vi "Reporte.vi"(10 "End Time":timestamp, 11 "Start Time":timestamp) -> ()   [LabVIEW 2020, in "UI.lvlib"]
uses:
  UI.lvlib
  Contabilidad/Contabilidad.lvlib
panel:
  out "Result Set":string[][](table) caption="Table Servicios"
  out "Tabla Servicios":string[](array[string])
  out "Ganacia Total":dbl
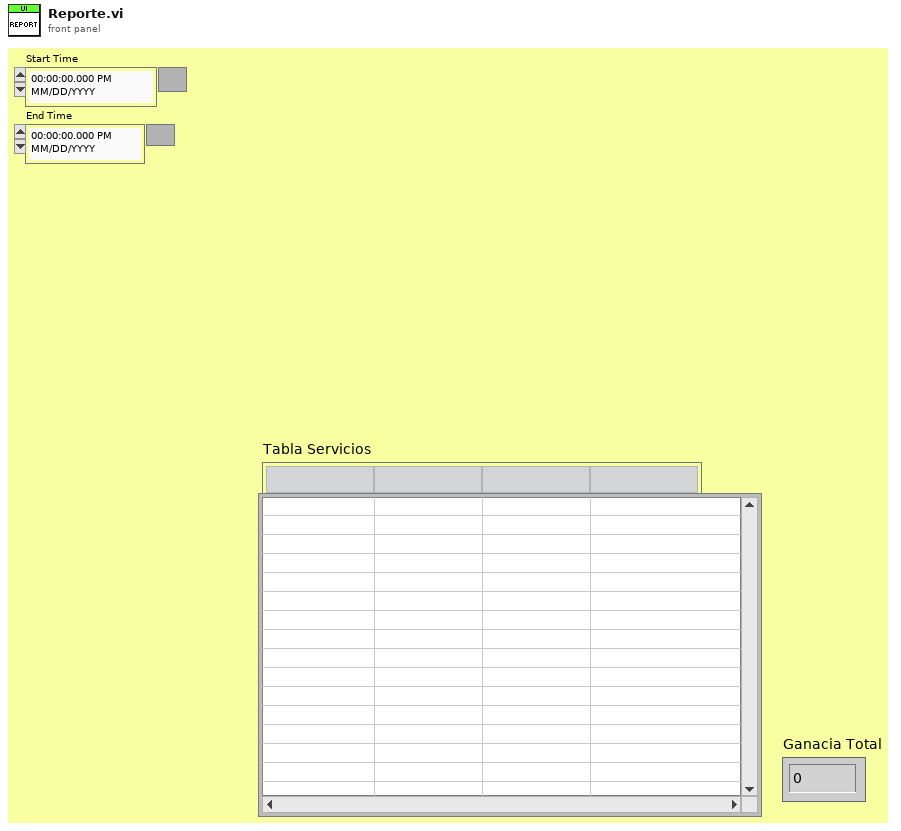
[diagram p1: front panel]
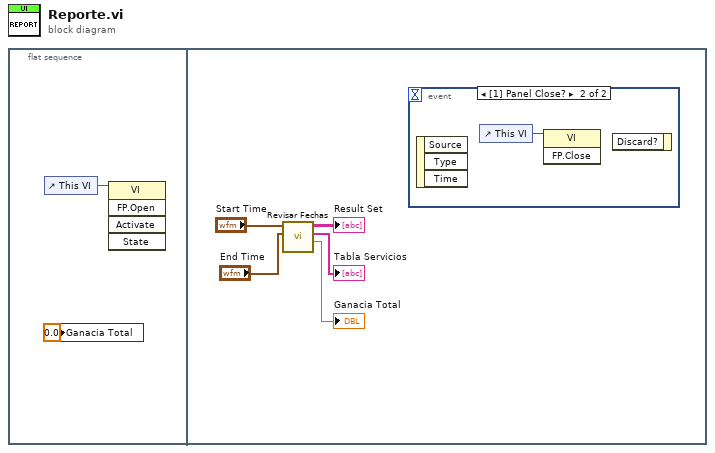
[diagram p0: block diagram]
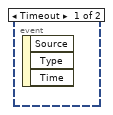
[diagram p2: hidden frame]
diagram:
  n1 = flat-sequence {
    frame #0 {
      n2 = control-ref of="This VI"() -> (w2:refnum<vi>)
      n3 = local write "Ganacia Total"(0.0 ("Suma")) -> ()
      n4 = invoke class="VI" method="FP.Open"(reference=w2) -> ()  [unwired: 4 in, 5 out]
    }
    frame #1 {
      n5 = call "Revisar Fechas.vi"("End Time"="End Time", "Start Time"="Start Time") -> ("Suma"=→"Ganacia Total":dbl, "Column Names"=→"Tabla Servicios":string[], "Result Set"=→"Result Set":string[][])  [unwired: 6 in, 1 out]
      n6 = event shown="[1] Panel Close?" {
        selector: _ -> [_ _]
        dyn-events: _ -> [_ _]
        timeout: _ -> [_ _]
        event Timeout {
          n7 = event-data() -> ()  [unwired: 1 in, 3 out]
        }
        event Panel Close? {
          n8 = event-data() -> ()  [unwired: 1 in, 3 out]
          n9 = control-ref of="This VI"() -> (w8:refnum<vi>)
          n10 = invoke class="VI" method="FP.Close"(reference=w8) -> ()  [unwired: 2 in, 3 out]
          n11 = event-data() -> ()  [unwired: 2 in, 1 out]
        }
      }
    }
  }
